vi "DT_Find Next Triangulation_Init.vi"(6 "next triangle in":i32, 7 "cur point":i32, 10 "Triangles In":i32[][](array[numeric]), 11 "Points In":cluster{"x":dbl, "y":dbl, "index":i32}[](array[cluster])) -> (0 "error":i32, 1 "Data":T1, 2 "Triangles Out":i32[][](array[numeric]), 3 "Points Out":cluster{"x":dbl, "y":dbl, "index":i32}[](array[cluster]), 4 "next triangle out":i32)   [LabVIEW 2017, in "NI_AAL_Geometry.lvlib"]
uses:
  <vilib>/Analysis/NI_AAL_Geometry.lvlib
  <vilib>/Analysis/geometry.llb/DT_Find Next Triangulation_Data.ctl
  <vilib>/Analysis/geometry.llb/DT_Triangle Manager_Get Oppo Point_in Ghost.vi
  <vilib>/Analysis/geometry.llb/DT_Triangle Manager_Get Global Point Index.vi
  <vilib>/Analysis/geometry.llb/DT_Triangle Manager_Get Adj_by Edge.vi
  <vilib>/Analysis/geometry.llb/DT_Triangle Manager_Get Oppo Point.vi
  <vilib>/Analysis/geometry.llb/DT_Triangle Manager_Get Ghost Point.vi
  <vilib>/Analysis/geometry.llb/DT_Triangle Manager_Get Adj_by Point.vi
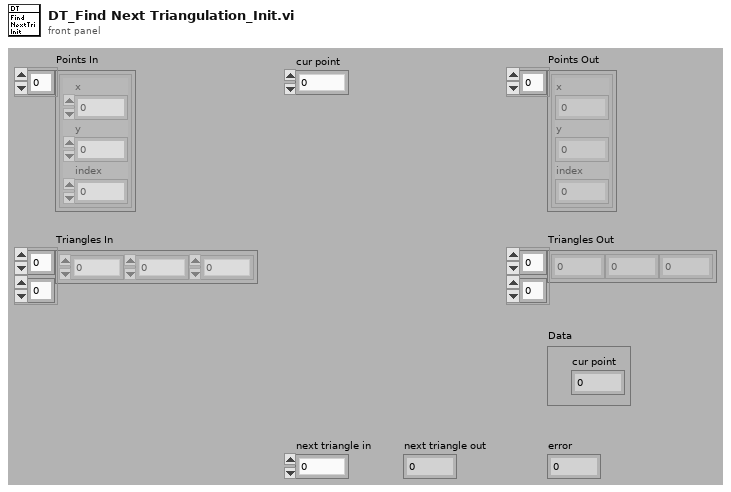
[diagram p1: front panel]
types:
  T1 = typedef "NI_AAL_Geometry.lvlib/DT_Find Next Triangulation_Data.ctl" = cluster{"cur point":i32, "cur triangle":i32, "cur local idx":i32, "base point":i32, "base triangle":i32, "base local idx":i32, "Candidate Triangles":i32[], "Candidate Point Idx":i32[]}
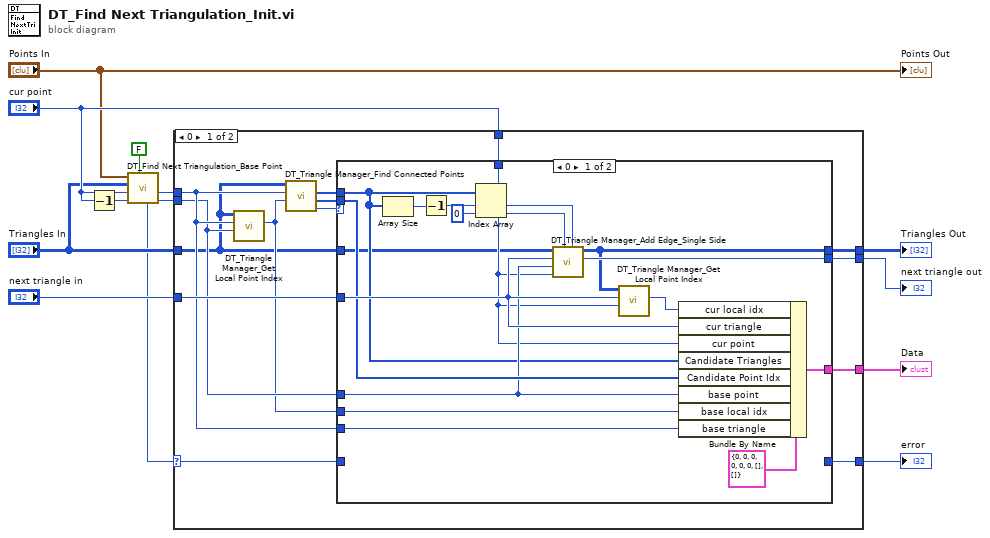
[diagram p0: block diagram]
diagram:
  n1 = Decrement(x="cur point") -> (x-1=w6:i32)
  n2 = call <vilib>:"DT_Find Next Triangulation_Base Point.vi"("left/right pt (right:F)"=FALSE, "search point"=w6, "external point"="cur point", "Triangles In"="Triangles In", "Points In"="Points In") -> ("base point"=w8:i32, "triangle"=w9:i32, "error"=w2:i32)  [unwired: 4 out]
  n3 = case shown="0" w2 {
    selector: w2 -> [w15 _]
    tunnel: [w27 _] -> w13
    tunnel: [w26 _] -> w12
    tunnel: [w25 _] -> w11
    tunnel: "next triangle in" -> [w24 _]
    tunnel: w9 -> [w22 _]
    tunnel: w8 -> [w21 _]
    tunnel: "cur point" -> [w19 _]
    tunnel: "Triangles In" -> [w17 _]
    tunnel: [w14 _] -> w1
    frame 0 {
      n4 = call <vilib>:"DT_Triangle Manager_Get Local Point Index.vi"("global idx"=w21, "triangle"=w22, "Triangles"=w17) -> ("local idx"=w20:i32)  [unwired: 8 out]
      n5 = call <vilib>:"DT_Triangle Manager_Find Connected Points.vi"("base point idx"=w20, "triangle"=w22, "Triangles"=w17) -> ("error"=w16:i32, "Connected Point Idx"=w23:i32[], "Connected Triangles"=w18:i32[])  [unwired: 6 out]
      n6 = case shown="0" w16 {
        selector: w16 -> [_ w46]
        tunnel: [w45 _] -> w27
        tunnel: [w43 _] -> w26
        tunnel: [w42 _] -> w25
        tunnel: w24 -> [w40 _]
        tunnel: w23 -> [w39 _]
        tunnel: w22 -> [w38 _]
        tunnel: w21 -> [w37 _]
        tunnel: w20 -> [w36 _]
        tunnel: w19 -> [w34 _]
        tunnel: w18 -> [w33 _]
        tunnel: w17 -> [w28 _]
        tunnel: w15 -> [_ _]
        tunnel: [_ w46] -> w14
        frame 0 {
          n7 = Array Size(array=w33) -> (size(s)=w32:i32)
          n8 = Decrement(x=w32) -> (x-1=w31:i32)
          n9 = Index Array(array=w33, index #1=w31, index #2=0 ("index")) -> (element #1=w35:i32, element #2=w30:i32)
          n10 = call <vilib>:"DT_Triangle Manager_Add Edge_Single Side.vi"("left bottom tri"=w35, "left top tri"=w30, "right point"=w34, "left point"=w37, "next triangle in"=w40, "Triangles In"=w28) -> ("next triangle out"=w45:i32, "Triangles Out"=w42:i32[][])  [unwired: 4 out]
          n11 = call <vilib>:"DT_Triangle Manager_Get Local Point Index.vi"("global idx"=w34, "triangle"=w40, "Triangles"=w42) -> ("local idx"=w41:i32)  [unwired: 8 out]
          n12 = Bundle By Name(cluster=T1 {"cur point"=0, "cur triangle"=0, "cur local idx"=0, "base point"=0, "base triangle"=0, "base local idx"=0, "Candidate Triangles"=[], "Candidate Point Idx"=[]} ("Data"), "cur local idx"=w41, "cur triangle"=w40, "cur point"=w34, "Candidate Triangles"=w33, "Candidate Point Idx"=w39, "base point"=w37, "base local idx"=w36, "base triangle"=w38) -> (w43:T1)
        }
        frame Default {
        }
      }
    }
    frame Default {
    }
  }
  "Triangles Out" <- w11
  "next triangle out" <- w13
  "Data" <- w12
  "error" <- w1
  "Points Out" <- "Points In"
